vi "Initialize Front Panel.vi"(8 "error in (no error)":errorcluster, 11 "For Loop Dialog in":refnum<class "Test Step Dialog.lvclass">) -> (0 "error out":errorcluster, 3 "For Loop Dialog out":refnum<class "Test Step Dialog.lvclass">)   [LabVIEW 2017, in "Test Step Dialog.lvclass"]
doc: "<License>\nCopyright © 2017 Composed Systems, LLC | All rights reserved\nwww.composed.io\n\nAuthor: Ethan Stern <ethan.stern@composed.io>\n\nThis software is provided \"AS IS\" WITHOUT WARRANTIES, either express or implied, AND IS FOR EDUCATIONAL PURPOSES ONLY.\n</License>"
uses:
  Test Step Dialog.lvclass
  Test Step Dialog.lvclass/Test Step Dialog.ctl
  ITest Executive Builder Dialog/ITest Executive Builder Dialog.lvclass
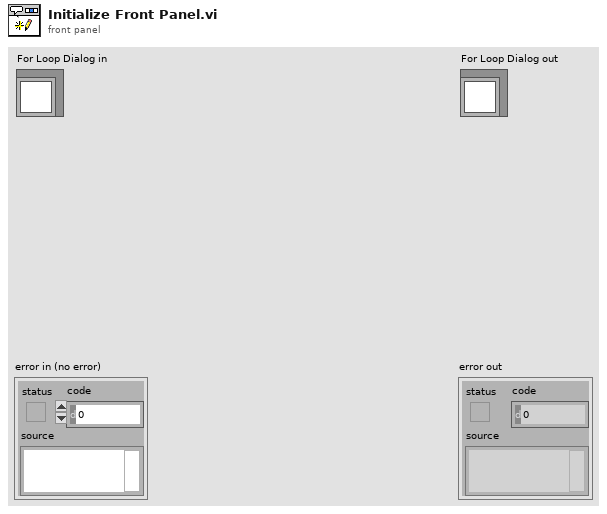
[diagram p1: front panel]
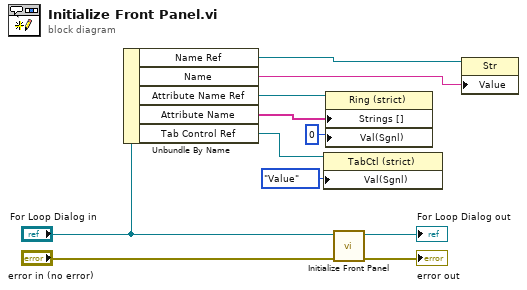
[diagram p0: block diagram]
diagram:
  n1 = Unbundle By Name("For Loop Dialog in") -> ("Name Ref"=w7:refnum<vi>, "Name"=w6:string, "Attribute Name Ref"=w5:refnum<vi>, "Attribute Name"=w4:string[], "Tab Control Ref"=w2:refnum<vi>)
  n2 = property class="TabCtl (strict)"(reference=w2, "Val(Sgnl)"=enum32{"Value", "Pointer"}."Value" ("Value (Signaling)")) -> ()  [unwired: 1 in, 2 out]
  n3 = property class="Ring (strict)"(reference=w5, "Strings []"=w4, "Val(Sgnl)"=u16 0 ("Value (Signaling)")) -> ()  [unwired: 1 in, 2 out]
  n4 = call-parent "Initialize Front Panel.vi"("error in (no error)"="error in (no error)", "ITest Executive Builder Dialog in"="For Loop Dialog in") -> ("error out"=→"error out":errorcluster, "ITest Executive Builder Dialog out"=→"For Loop Dialog out":refnum<class "Test Step Dialog.lvclass">)  [unwired: 8 in]
  n5 = property class="Str"(reference=w7, "Value"=w6) -> ()  [unwired: 1 in, 2 out]
